vi "第二題.vi"() -> ()   [LabVIEW 2019]
panel:
  out "Waveform Chart":cluster{dbl, dbl}(graph)
  in  "Stop":bool
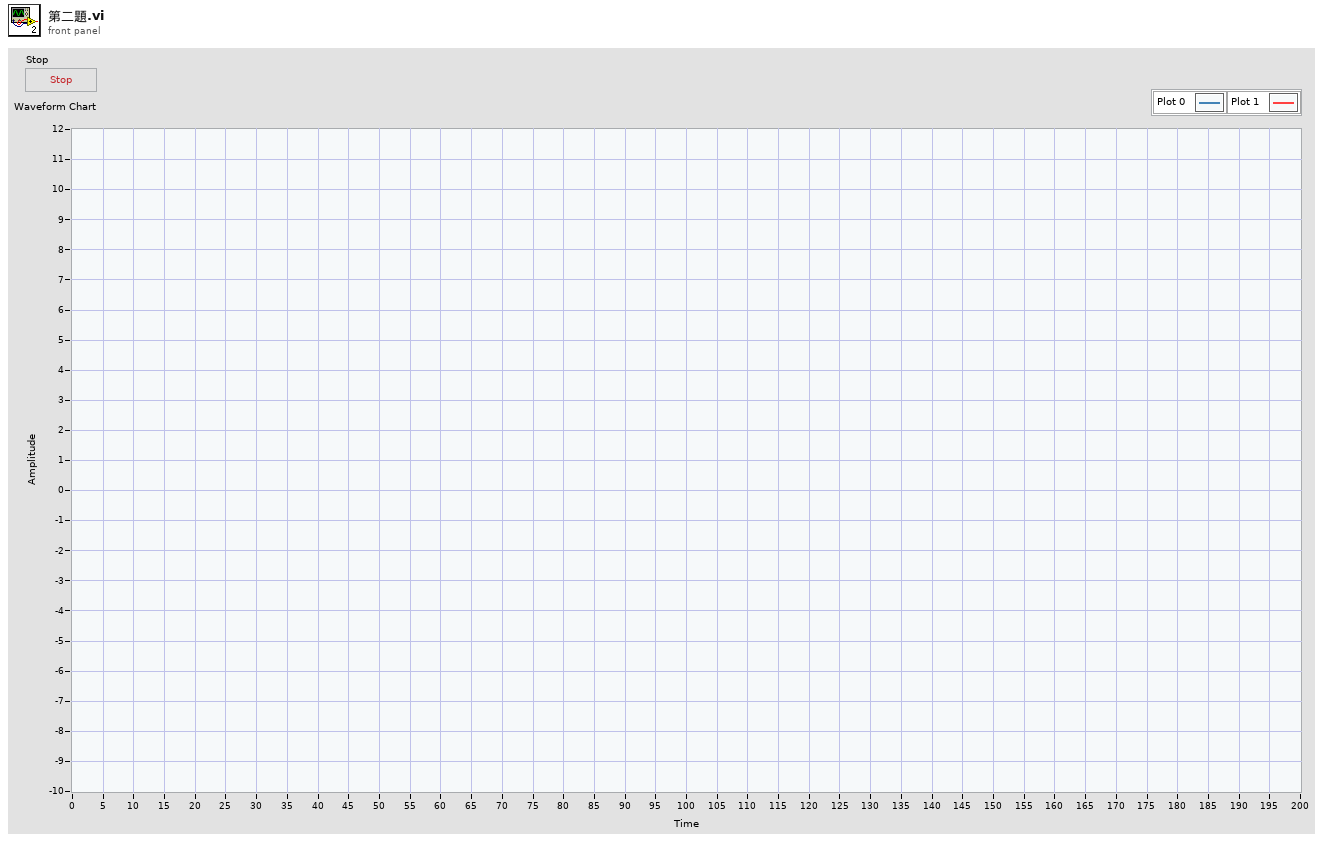
[diagram p1: front panel]
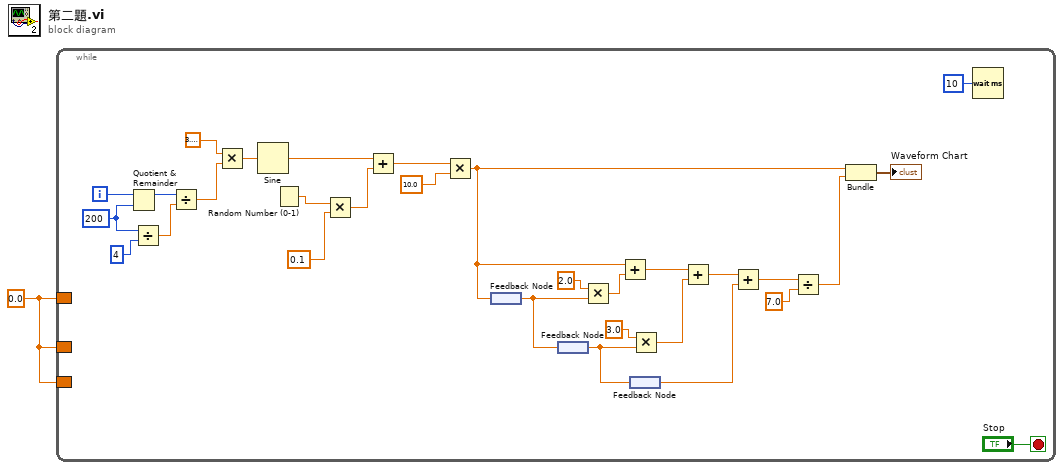
[diagram p0: block diagram]
diagram:
  w1 = 0.0
  n1 = while {
    border: w1 -> [_]
    border: w1 -> [_]
    border: w1 -> [_]
    i -> [w20]
    stop <- "Stop" stop-if-true
    w18 = 200
    n2 = Quotient & Remainder(x=w20, y=w18) -> (x-y*floor(x/y)=w19:i32)  [unwired: 1 out]
    n3 = Divide(x=w18, y=4) -> (x/y=w16:dbl)
    n4 = Divide(x=w19, y=w16) -> (x/y=w25:dbl)
    n5 = Multiply(x=3.141592653589793, y=w25) -> (x*y=w26:dbl)
    n6 = Sine(x=w26) -> (sin(x)=w24:dbl)
    n7 = Random Number (0-1)() -> (number: 0 to 1=w23:dbl)
    n8 = Multiply(x=w23, y=0.1) -> (x*y=w22:dbl)
    n9 = Add(x=w24, y=w22) -> (x+y=w31:dbl)
    n10 = Multiply(x=w31, y=10.0) -> (x*y=w6:dbl)
    n11 = feedback-in #1(w6) -> ()
    n12 = feedback #1() -> (w11:dbl)
    n13 = feedback #2() -> (w8:dbl)
    n14 = feedback-in #2(w11) -> ()
    n15 = Multiply(x=2.0, y=w11) -> (x*y=w15:dbl)
    n16 = Add(x=w6, y=w15) -> (x+y=w13:dbl)
    n17 = feedback #3() -> (w7:dbl)
    n18 = feedback-in #3(w8) -> ()
    n19 = Multiply(x=3.0, y=w8) -> (x*y=w10:dbl)
    n20 = Add(x=w13, y=w10) -> (x+y=w9:dbl)
    n21 = Add(x=w9, y=w7) -> (x+y=w4:dbl)
    n22 = Divide(x=w4, y=7.0) -> (x/y=w2:dbl)
    n23 = Bundle(w6, w2) -> (→"Waveform Chart":cluster{dbl, dbl})  [unwired: 1 in]
    n24 = Wait (ms)(milliseconds to wait=u32 10) -> ()  [unwired: 1 out]
  }
